vi "Preview the image.vi"() -> ()   [LabVIEW 2009]
uses:
  D/Program Files (x86)/National Instruments/LabVIEW 2015/user.lib/LabViewDVPCamera/LabViewDVPCamera.lvlib
panel:
  out "Image":T1(plugin-control)
  in  "CloseFlg":i32
  out "handle":u32
  in  "CameraList":u16(ring) items=["USB2_1.2M_MONO(31)@UE121000026", "USB3_CMOS_16M(2)@UB16A000000"]
  in  "Set":bool
  in  "Close":bool
  in  "Open":bool
  in  "ScanCamera":bool
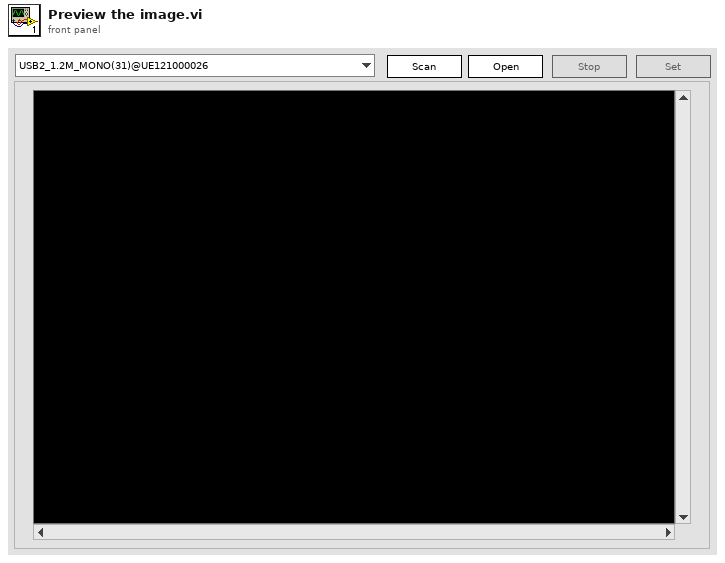
[diagram p1: front panel]
types:
  T1 = typedef "IMAQ Image.ctl" = refnum<image>
  T2 = enum8{"Enabled", "Disabled", "Disabled and Grayed Out"}
  T3 = typedef "LVStringsAndValuesArrayTypeDef_U16.ctl" = cluster{"String":string, "Value":u16}[]
  T4 = typedef "Image Type" = u32
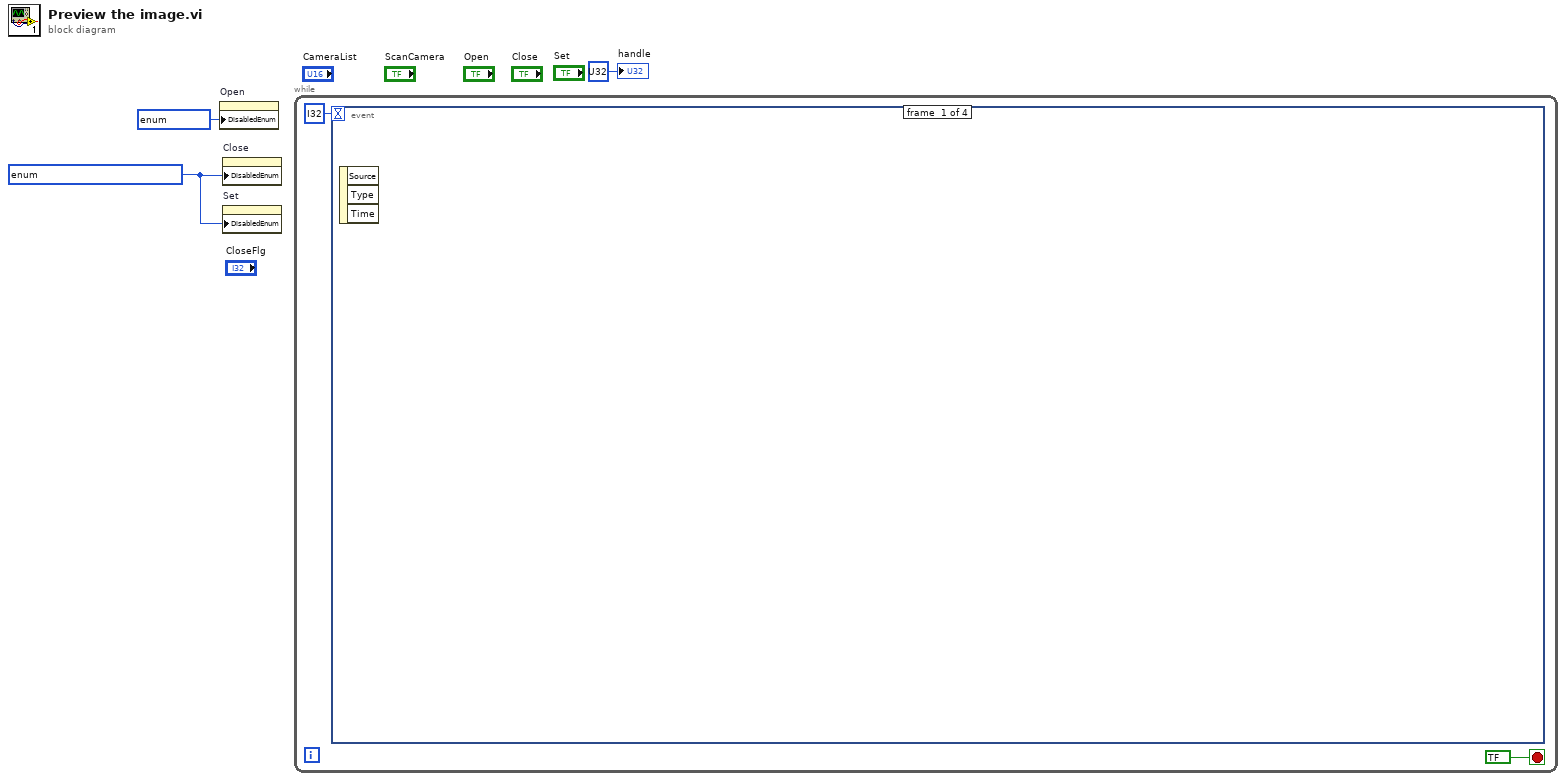
[diagram p0: block diagram]
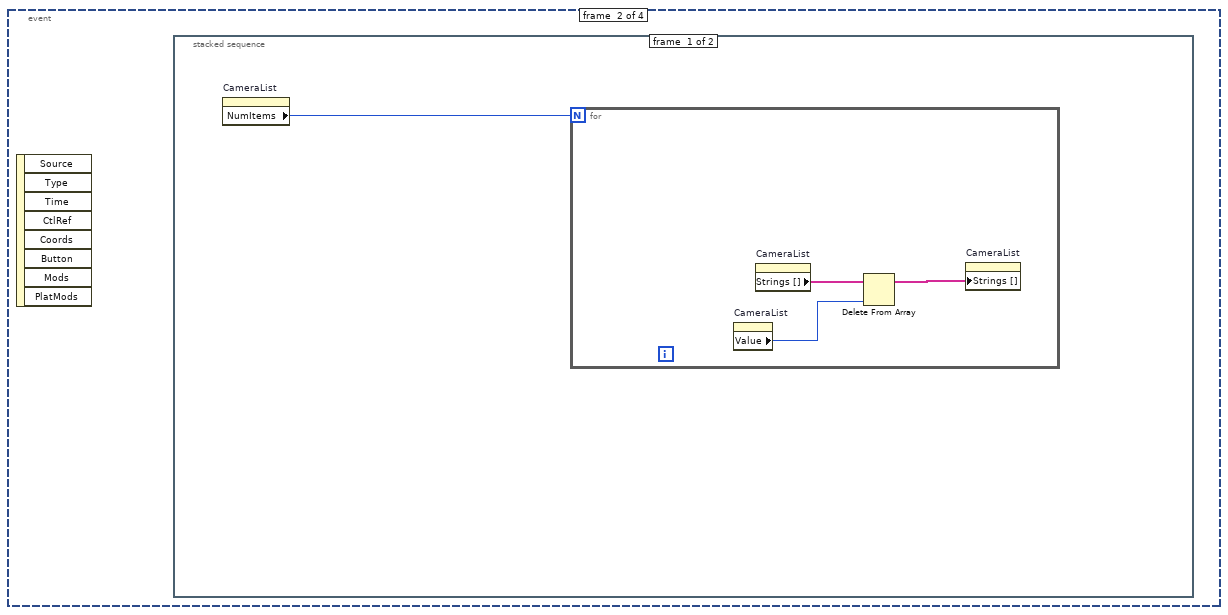
[diagram p2: hidden frame]
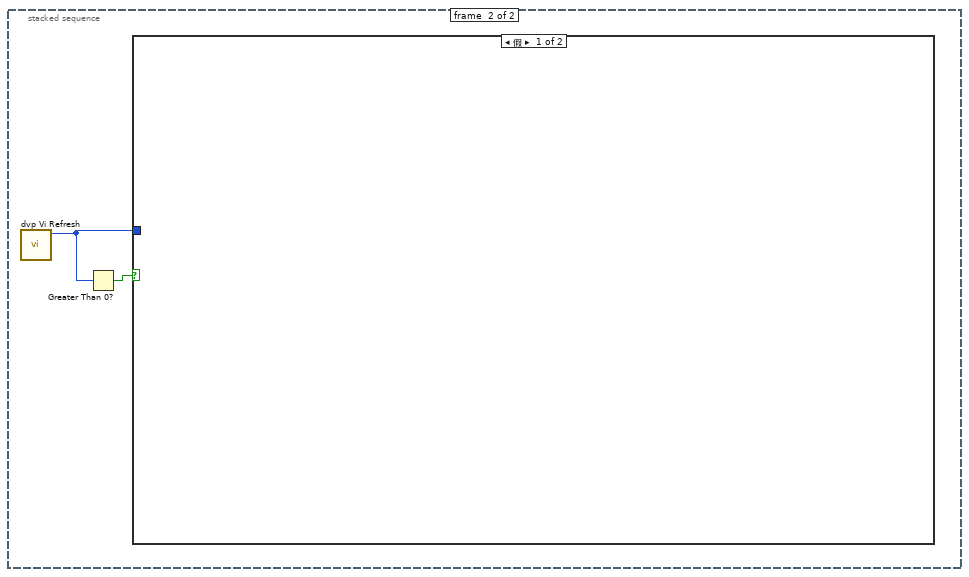
[diagram p3: hidden frame]
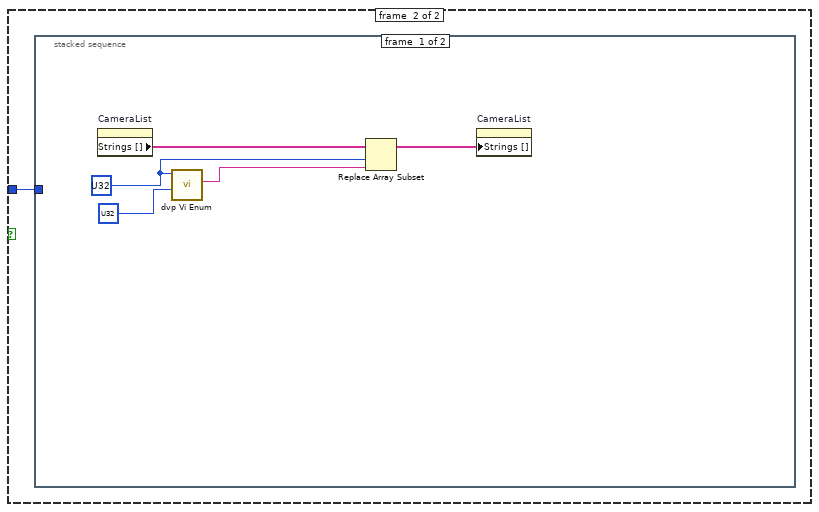
[diagram p4: hidden frame]
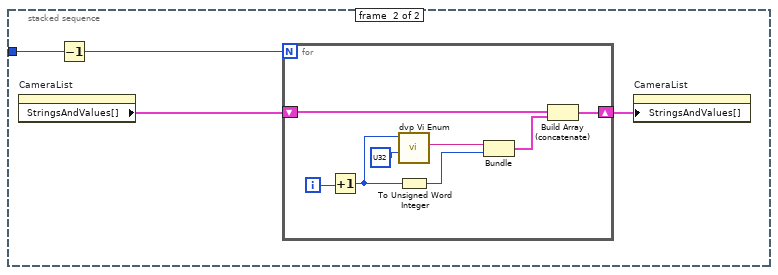
[diagram p5: hidden frame]
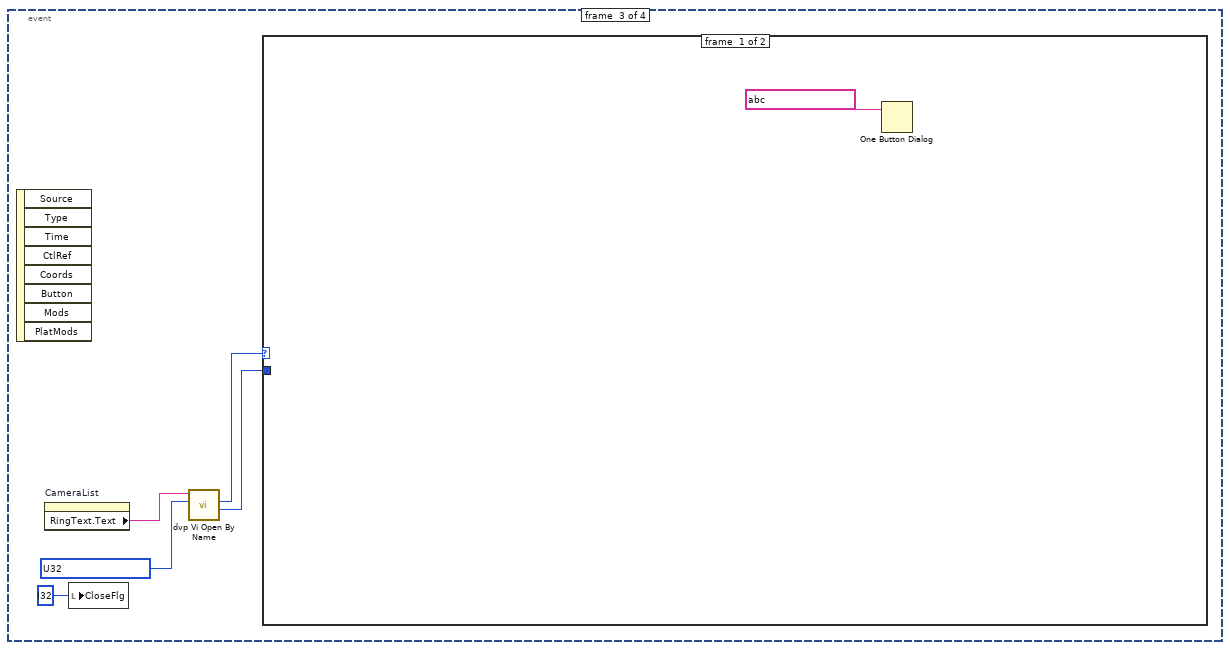
[diagram p6: hidden frame]
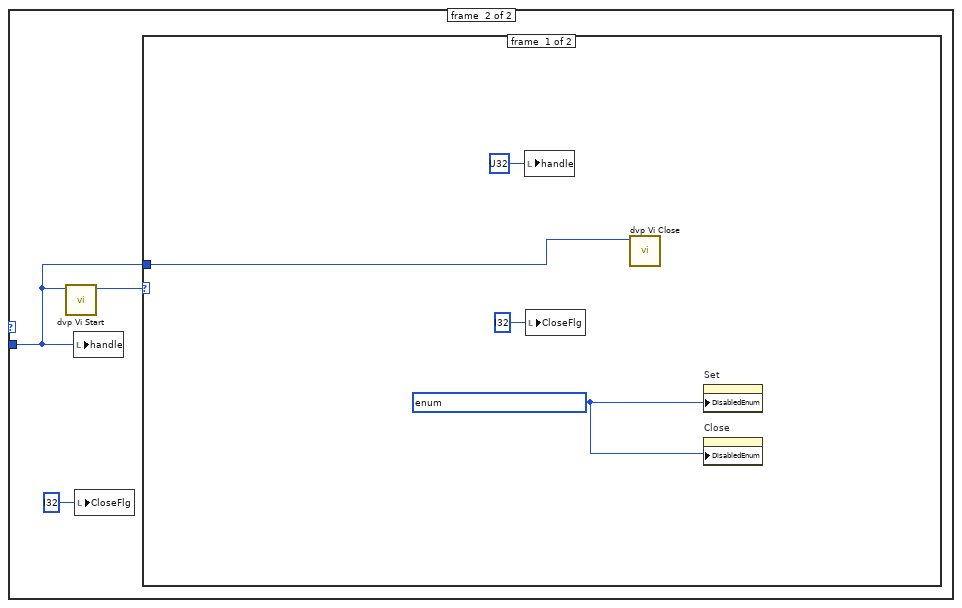
[diagram p7: hidden frame]
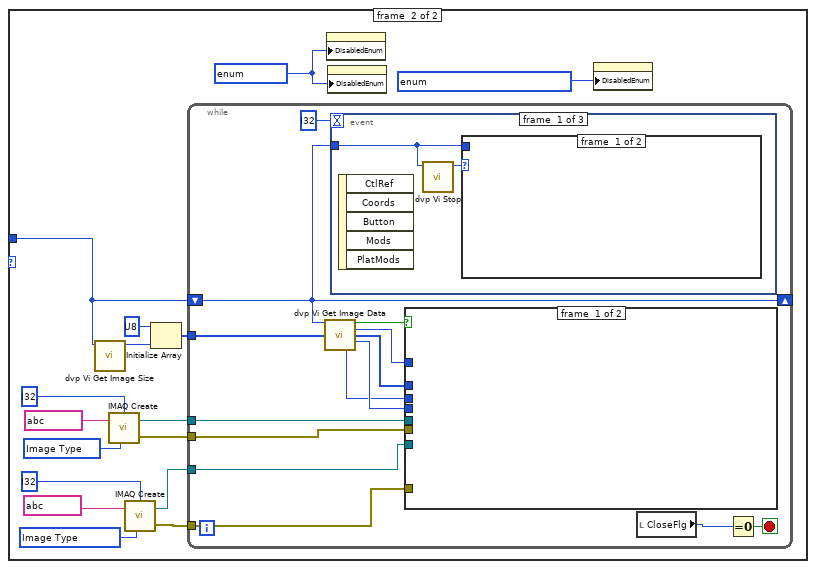
[diagram p8: hidden frame]
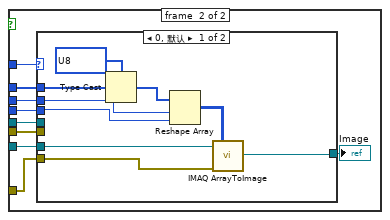
[diagram p9: hidden frame]
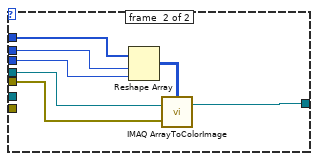
[diagram p10: hidden frame]
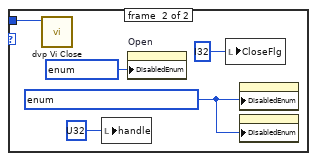
[diagram p11: hidden frame]
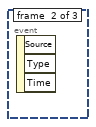
[diagram p12: hidden frame]
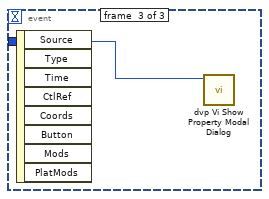
[diagram p13: hidden frame]
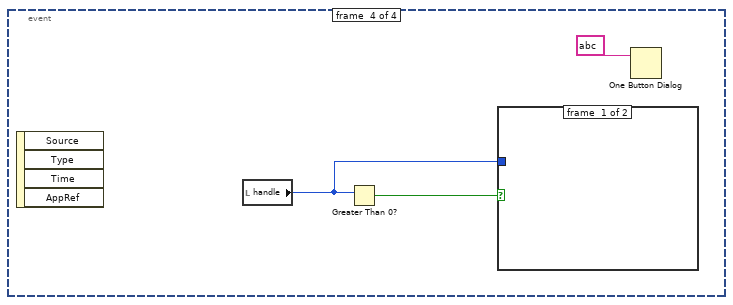
[diagram p14: hidden frame]
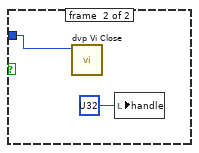
[diagram p15: hidden frame]
diagram:
  w2 = T2 ? ("禁用")
  n1 = property on="Open" class="Bool"("DisabledEnum"=T2 ? ("禁用")) -> ()  [unwired: 2 in, 2 out]
  n2 = property on="Close" class="Bool"("DisabledEnum"=w2) -> ()  [unwired: 2 in, 2 out]
  n3 = property on="Set" class="Bool"("DisabledEnum"=w2) -> ()  [unwired: 2 in, 2 out]
  n4 = while {
    stop <- bool ? stop-if-true
    n5 = event shown="[2] \"Open\": 鼠标按下" {
      selector: _ -> [_ _ _ _]
      dyn-events: _ -> [_ _ _ _]
      timeout: i32 ? -> [_ _ _ _]
      event #0 {
        n6 = event-data() -> ()  [unwired: 1 in, 3 out]
      }
      event #1 {
        n7 = event-data() -> ()  [unwired: 1 in, 8 out]
        n8 = stacked-sequence "清除下拉列表的数据" {
          frame #0 {
            n9 = property on="CameraList" class="Ring (严格)"() -> ("NumItems"=w6:u32)  [unwired: 2 in, 2 out]
            n10 = for {
              N: w6 -> [_]
              n11 = property on="CameraList" class="Ring (严格)"() -> ("Value"=w8:u16)  [unwired: 2 in, 2 out]
              n12 = property on="CameraList" class="Ring (严格)"() -> ("Strings []"=w7:string[])  [unwired: 2 in, 2 out]
              n13 = Delete From Array ("删除数组元素")(array=w7, index=w8) -> (array with subset deleted=w9:string[])  [unwired: 1 in, 1 out]
              n14 = property on="CameraList" class="Ring (严格)"("Strings []"=w9) -> ()  [unwired: 2 in, 2 out]
            }
          }
          frame #1 {
            n15 = call "dvp Vi Refresh.vi"() -> ("pCount out"=w11:u32)  [unwired: 10 in, 1 out]
            n16 = Greater Than 0?(x=w11) -> (x > 0?=w10:bool)
            n17 = case shown="假" w10 {
              tunnel: w11 -> [_ w12]
              frame #0 {
              }
              frame #1 {
                n18 = stacked-sequence {
                  tunnel: w12 -> [_ w19]
                  frame #0 {
                    w13 = u32 ? ("index")
                    n19 = property on="CameraList" class="Ring (严格)"() -> ("Strings []"=w16:string[])  [unwired: 2 in, 2 out]
                    n20 = call "dvp Vi Enum.vi"("unSize"=u32 ?, "index"=w13) -> ("friendlyName out"=w15:string)  [unwired: 8 in, 1 out]
                    n21 = Replace Array Subset ("替换数组子集")(array=w16, new element=w15, index=w13) -> (w17:string[])
                    n22 = property on="CameraList" class="Ring (严格)"("Strings []"=w17) -> ()  [unwired: 2 in, 2 out]
                  }
                  frame #1 {
                    n23 = property on="CameraList" class="Ring (严格)"() -> ("StringsAndValues[]"=w21:T3)  [unwired: 2 in, 2 out]
                    n24 = Decrement(x=w19) -> (x-1=w18:u32)
                    n25 = for {
                      N: w18 -> [_]
                      shift-right: [w28] -> w20
                      shift-left: w21 -> [w26]
                      i -> [w23]
                      n26 = Increment(x=w23) -> (x+1=w22:i32)
                      n27 = call "dvp Vi Enum.vi"("unSize"=u32 ?, "index"=w22) -> ("friendlyName out"=w29:string)  [unwired: 8 in, 1 out]
                      n28 = To Unsigned Word Integer(number=w22) -> (unsigned 16bit integer=w25:u16)
                      n29 = Bundle("friendlyName out"=w29, w25) -> (w27:cluster{"friendlyName out":string, u16})  [unwired: 1 in]
                      n30 = Build Array (concatenate) ("创建数组")(w26, w27) -> (w28:T3)
                    }
                    n31 = property on="CameraList" class="Ring (严格)"("StringsAndValues[]"=w20) -> ()  [unwired: 2 in, 2 out]
                  }
                }
              }
            }
          }
        }
      }
      event #2 {
        w32 = u32 ? items=["OPEN_OFFLINE", "OPEN_NORMAL"] ("type")
        n32 = event-data() -> ()  [unwired: 1 in, 8 out]
        n33 = property on="CameraList" class="Ring (严格)"() -> ("RingText.Text"=w31:string)  [unwired: 2 in, 2 out]
        n34 = local write "CloseFlg"(i32 ? ("CloseFlg")) -> ()
        n35 = call "dvp Vi Open By Name.vi"("type"=w32, "friendlyName"=w31) -> ("pHandle out"=w34:u32, "function return"=w33:u32)  [unwired: 7 in, 1 out]
        n36 = case shown="1" w33 {
          tunnel: w34 -> [_ w38]
          frame #0 {
            n37 = One Button Dialog(message=string ? ("消息")) -> ()  [unwired: 1 in, 1 out]
          }
          frame #1 {
            n38 = call "dvp Vi Start.vi"("handle"=w38) -> ("function return"=w36:u32)  [unwired: 10 in]
            n39 = local write "handle"(w38) -> ()
            n40 = local write "CloseFlg"(i32 ? ("CloseFlg")) -> ()
            n41 = case shown="1" w36 {
              tunnel: w38 -> [w42 w54]
              frame #0 {
                w41 = T2 ? ("禁用")
                n42 = local write "handle"(u32 ? ("handle")) -> ()
                n43 = local write "CloseFlg"(i32 ? ("CloseFlg")) -> ()
                n44 = call "dvp Vi Close.vi"("handle"=w42) -> ()  [unwired: 10 in, 1 out]
                n45 = property on="Set" class="Bool"("DisabledEnum"=w41) -> ()  [unwired: 2 in, 2 out]
                n46 = property on="Close" class="Bool"("DisabledEnum"=w41) -> ()  [unwired: 2 in, 2 out]
              }
              frame #1 {
                w49 = T4 ? items=["Grayscale (U8)", "Grayscale (I16)", "Grayscale (SGL)", "Complex (CSG)", "RGB (U32)", "HSL (U32)", "RGB (U64)", "Grayscale (U16)"] ("Image Type")
                w52 = T4 ? items=["Grayscale (U8)", "Grayscale (I16)", "Grayscale (SGL)", "Complex (CSG)", "RGB (U32)", "HSL (U32)", "RGB (U64)", "Grayscale (U16)"] ("Image Type")
                w58 = T2 ? ("禁用")
                n47 = call "dvp Vi Get Image Size.vi"("handle"=w54) -> ("function return"=w53:u32)  [unwired: 10 in]
                n48 = call "IMAQ Create"("Border Size"=i32 ?, "Image Name"=string ?, "Image Type"=w49) -> ("New Image"=w47:T1, "error out"=w46:errorcluster)  [unwired: 2 in]
                n49 = call "IMAQ Create"("Border Size"=i32 ?, "Image Name"=string ?, "Image Type"=w52) -> ("New Image"=w44:T1, "error out"=w43:errorcluster)  [unwired: 2 in]
                n50 = Initialize Array(u8 ? ("元素"), w53) -> (w55:u8[])
                n51 = while {
                  shift-right: [w69] -> _
                  shift-left: w54 -> [w69]
                  tunnel: w55 -> [w68]
                  tunnel: w47 -> [w62]
                  tunnel: w46 -> [w61]
                  tunnel: w44 -> [w59]
                  tunnel: w43 -> [w60]
                  stop <- w71 stop-if-true
                  n52 = call "dvp Vi Get Image Data.vi"("handle"=w69, "pbuffer"=w68) -> ("piHeight out"=w66:i32, "function return"=w63:bool, "pformat out"=w64:i32, "pbuffer out"=w65:u32[], "piWidth out"=w67:i32)  [unwired: 9 in]
                  n53 = event shown="[1] 超时" {
                    selector: _ -> [_ _ _]
                    dyn-events: _ -> [_ _ _]
                    timeout: i32 ? -> [_ _ _]
                    tunnel: w69 -> [w98 _ w105]
                    event #0 {
                      n54 = event-data() -> ()  [unwired: 1 in, 5 out]
                      n55 = call "dvp Vi Stop.vi"("handle"=w98) -> ("function return"=w99:u32)  [unwired: 10 in]
                      n56 = case shown="1" w99 {
                        tunnel: w98 -> [_ w102]
                        frame #0 {
                        }
                        frame #1 {
                          w101 = T2 ? ("禁用")
                          n57 = call "dvp Vi Close.vi"("handle"=w102) -> ()  [unwired: 10 in, 1 out]
                          n58 = local write "handle"(u32 ? ("handle")) -> ()
                          n59 = property on="Open" class="Bool"("DisabledEnum"=T2 ? ("禁用")) -> ()  [unwired: 2 in, 2 out]
                          n60 = local write "CloseFlg"(i32 ? ("CloseFlg")) -> ()
                          n61 = property on="Close" class="Bool"("DisabledEnum"=w101) -> ()  [unwired: 2 in, 2 out]
                          n62 = property on="Set" class="Bool"("DisabledEnum"=w101) -> ()  [unwired: 2 in, 2 out]
                        }
                      }
                    }
                    event #1 {
                      n63 = event-data() -> ()  [unwired: 1 in, 3 out]
                    }
                    event #2 {
                      n64 = event-data() -> ()  [unwired: 1 in, 8 out]
                      n65 = call "dvp Vi Show Property Modal Dialog.vi"("handle"=w105) -> ()  [unwired: 10 in, 1 out]
                    }
                  }
                  n66 = case shown="真" w63 {
                    tunnel: w67 -> [_ w81]
                    tunnel: w66 -> [_ w80]
                    tunnel: w65 -> [_ w78]
                    tunnel: w64 -> [_ w77]
                    tunnel: w62 -> [_ w75]
                    tunnel: w61 -> [_ w74]
                    tunnel: w60 -> [_ w73]
                    tunnel: w59 -> [_ w76]
                    frame #0 {
                    }
                    frame #1 {
                      n67 = case shown="0, 默认" w77 {
                        tunnel: w80 -> [w90 w96]
                        tunnel: w81 -> [w89 w97]
                        tunnel: [w88 w94] -> w79
                        tunnel: w78 -> [w85 w93]
                        tunnel: w76 -> [w82 _]
                        tunnel: w75 -> [_ w92]
                        tunnel: w74 -> [_ w91]
                        tunnel: w73 -> [w83 _]
                        frame #0 {
                          n68 = Type Cast(type=u8[] ?, x=w85) -> (*(type *) &x=w84:u8[])
                          n69 = Reshape Array ("重排数组维数")(w84, w90, w89) -> (w87:u8[][])
                          n70 = call "IMAQ ArrayToImage"("error in (no error)"=w83, "Image Pixels (U8)"=w87, "Image"=w82) -> ("Image Out"=w88:T1)  [unwired: 7 in, 1 out]
                        }
                        frame #1 {
                          n71 = Reshape Array ("重排数组维数")(w93, w96, w97) -> (w95:u32[][])
                          n72 = call "IMAQ ArrayToColorImage"("Image Pixels (U32)"=w95, "Image"=w92, "error in (no error)"=w91) -> ("Image Out"=w94:T1)  [unwired: 2 in, 1 out]
                        }
                      }
                      "Image" <- w79
                    }
                  }
                  n73 = local read "CloseFlg"() -> (w70:i32)
                  n74 = Equal To 0?(x=w70) -> (x = 0?=w71:bool)
                }
                n75 = property on="Set" class="Bool"("DisabledEnum"=w58) -> ()  [unwired: 2 in, 2 out]
                n76 = property on="Close" class="Bool"("DisabledEnum"=w58) -> ()  [unwired: 2 in, 2 out]
                n77 = property on="Open" class="Bool"("DisabledEnum"=T2 ? ("禁用")) -> ()  [unwired: 2 in, 2 out]
              }
            }
          }
        }
      }
      event #3 {
        n78 = event-data() -> ()  [unwired: 1 in, 4 out]
        n79 = local read "handle"() -> (w106:u32)
        n80 = Greater Than 0?(x=w106) -> (x > 0?=w107:bool)
        n81 = case shown="真" w107 {
          tunnel: w106 -> [_ w110]
          frame #0 {
          }
          frame #1 {
            n82 = call "dvp Vi Close.vi"("handle"=w110) -> ()  [unwired: 10 in, 1 out]
            n83 = local write "handle"(u32 ? ("handle")) -> ()
          }
        }
        n84 = One Button Dialog(message=string ? ("消息")) -> ()  [unwired: 1 in, 1 out]
      }
    }
  }
  "handle" <- u32 ? ("handle")
